vi "Open.vi"(8 "Error In":errorcluster {"code" format="%.0x"}, 11 "IP Address":string="192.168.1.218") -> (0 "Error Out":errorcluster {"code" format="%.0x"}, 3 "Cards Out":cluster{"Session":u32, "Card number":u32}[](array[cluster]))   [LabVIEW 2012, in "Virtual-PGA.lvlib"]
doc: "This VI establishes communication with the switch."
uses:
  Virtual-PGA.lvlib
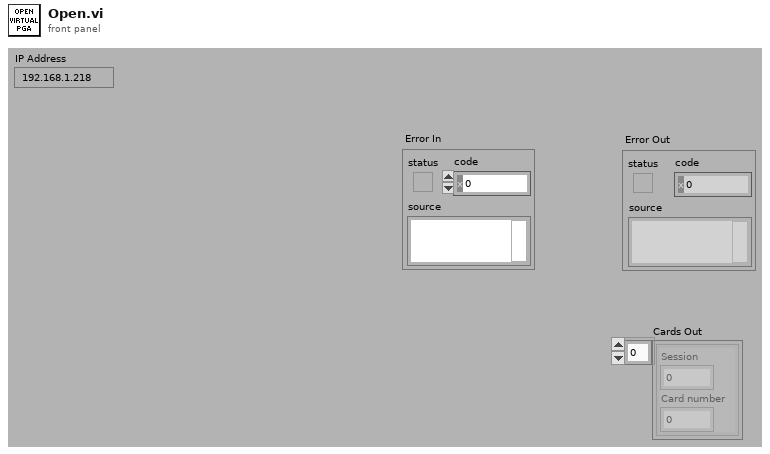
[diagram p1: front panel]
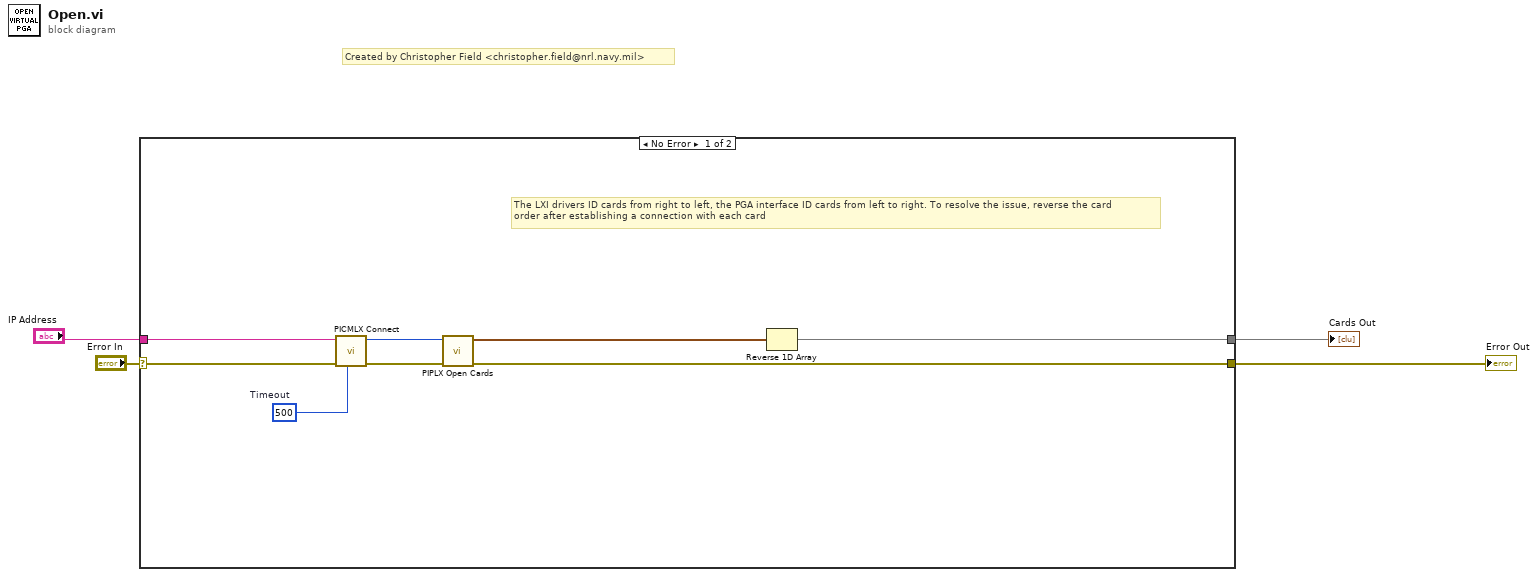
[diagram p0: block diagram]
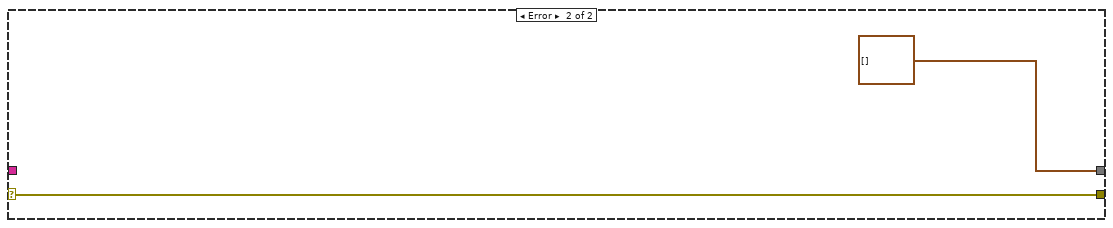
[diagram p2: hidden frame]
diagram:
  # "Created by Christopher Field <christopher.field@nrl.navy.mil>"
  n1 = case shown="No Error" "Error In" {
    selector: "Error In" -> [w11 w14]
    tunnel: [w5 cluster{"Session":u32, "Card number":u32}[] [] ("Output handles")] -> w4
    tunnel: [w8 w14] -> w3
    tunnel: "IP Address" -> [w7 _]
    frame No Error {
      w12 = u32 500  # Timeout
      # "The LXI drivers ID cards from right to left, the PGA interface ID cards from left to right. To resolve the issue, reverse the card\norder after establishing a connection with each card"
      n2 = call <instrlib>:"PICMLX Connect.vi"("Timeout"=w12, "error in"=w11, "Remote Machine"=w7) -> ("error out"=w9:errorcluster, "Session ID"=w10:u32)  [unwired: 6 in]
      n3 = call <instrlib>:"PIPLX Open Cards.vi"("error in"=w9, "Session"=w10) -> ("error out"=w8:errorcluster, "Output handles"=w6:cluster{"Session":u32, "Card number":u32}[])  [unwired: 7 in, 1 out]
      n4 = Reverse 1D Array(array=w6) -> (reversed array=w5:cluster{"Session":u32, "Card number":u32}[])
    }
    frame Error {
    }
  }
  "Error Out" <- w3
  "Cards Out" <- w4
